vi "Write_raw_block_header.vi"(2 "Block Timings":T1, 3 "No of PWA samples":i32, 4 "Add to Block Header":string) -> (5 "Output string":string)   [LabVIEW 2020]
uses:
  Globals/Meas_global.vi
  Globals/Plug_in_data_global.vi
  Controls/Block_start_and_end.ctl
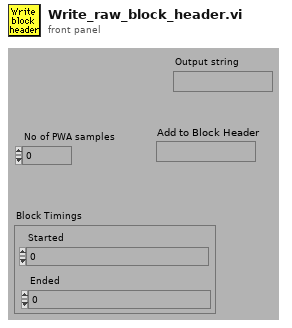
[diagram p1: front panel]
types:
  T1 = typedef "Block_start_and_end.ctl" = cluster{"Started":dbl, "Ended":dbl}
  T2 = typedef "Ch_description_ADAM.ctl" = cluster{"Ch Name":string, "Type":T3, "Function":T4, "Ch State":T5, "Calibration type":T6, "A":dbl, "B":dbl, "C":dbl, "D":dbl, "Comments":string, "Address":T7, "String":string, "Duty":u16}
  T3 = typedef "Module_type_ADAM.ctl" = string
  T4 = typedef "Function_ADAM.ctl" = enum16{"Analogue Input", "Digital Input", "Event counter", "Event rate", "Analogue Output", "Digital Output", "Relay Output"}
  T5 = typedef "Channel_State.ctl" = enum16{"On", "Off", "Always On", "Always Off"}
  T6 = typedef "Calib_type_ADAM.ctl" = string
  T7 = typedef "Address.ctl" = cluster{"Main":i32, "Ch.":i32, "Sub":i32, "Port Name":string}
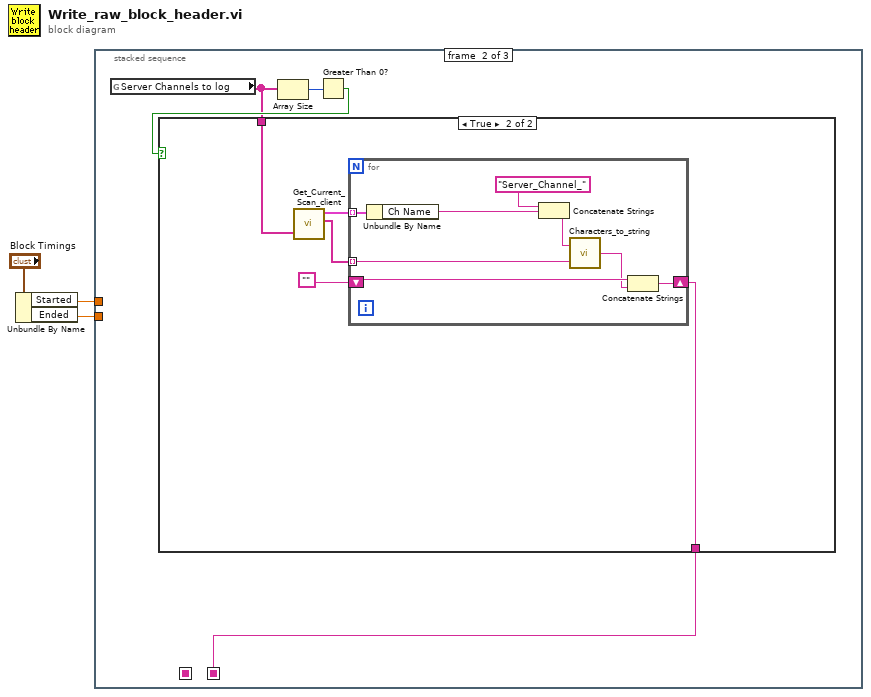
[diagram p0: block diagram]
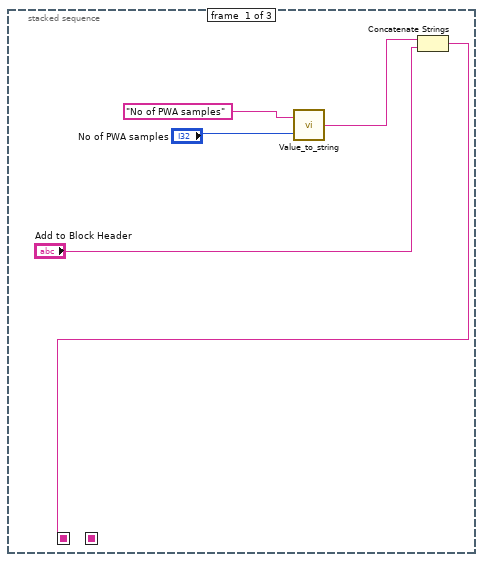
[diagram p2: hidden frame]
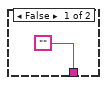
[diagram p3: hidden frame]
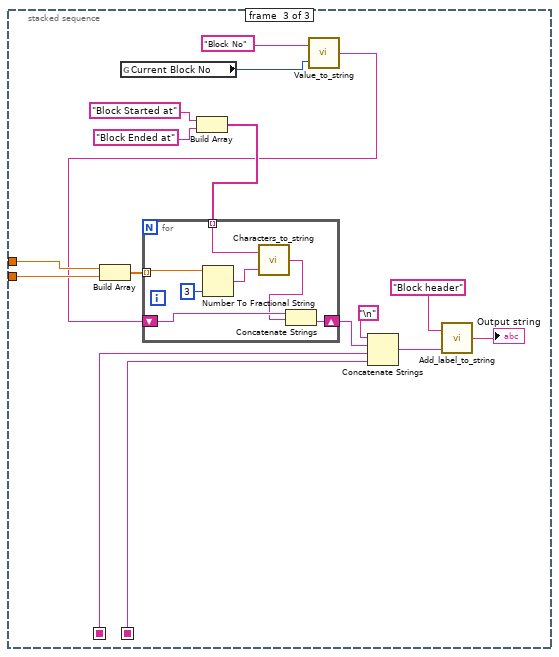
[diagram p4: hidden frame]
diagram:
  n1 = Unbundle By Name("Block Timings") -> ("Started"=w2:dbl, "Ended"=w1:dbl)
  n2 = stacked-sequence {
    seq-local: [w8 _ _] -> [_ _ w41]
    seq-local: [_ w9 _] -> [_ _ w28]
    tunnel: w2 -> [_ _ w34]
    tunnel: w1 -> [_ _ w33]
    frame #0 {
      n3 = call "Value_to_string.vi"("Value"="No of PWA samples", "Label for value"="No of PWA samples") -> ("Output string"=w5:string)  [unwired: 1 in]
      n4 = Concatenate Strings(w5, "Add to Block Header") -> (w8:string)
    }
    frame #1 {
      n5 = global read "Plug_in_data_global.vi" "Server Channels to log"() -> (w10:string[])
      n6 = Array Size(array=w10) -> (size(s)=w12:i32)
      n7 = Greater Than 0?(x=w12) -> (x > 0?=w11:bool)
      n8 = case shown="True" w11 {
        tunnel: w10 -> [_ w17]
        tunnel: ["" w14] -> w9
        frame False {
        }
        frame True {
          n9 = call "Get_Current_Scan_client.vi"("multipleChannels"=w17) -> ("Ch Description Array"=w16:T2[], "String values"=w15:string[])  [unwired: 2 in, 1 out]
          n10 = for {
            shift-right: [w25] -> w14
            shift-left: "" -> [w24]
            tunnel: w16 -> [w21] mode=indexing
            tunnel: w15 -> [w19] mode=indexing
            n11 = Unbundle By Name(w21) -> ("Ch Name"=w20:string)
            n12 = Concatenate Strings("Server_Channel_" ("string"), w20) -> (w22:string)
            n13 = call "Characters_to_string.vi"("Characters to write"=w19, "Label for characters"=w22) -> ("Output string"=w23:string)  [unwired: 1 in]
            n14 = Concatenate Strings(w24, w23) -> (w25:string)
          }
        }
      }
    }
    frame #2 {
      n15 = Build Array(w34, w33) -> (w35:dbl[])
      n16 = global read "Meas_global.vi" "Current Block No"() -> (w27:i32)
      n17 = Build Array("Block Started at", "Block Ended at") -> (w37:string[])
      n18 = call "Value_to_string.vi"("Value"=w27, "Label for value"="Block No") -> ("Output string"=w31:string)  [unwired: 1 in]
      n19 = for {
        tunnel: w37 -> [w49] mode=indexing
        shift-right: [w46] -> w39
        shift-left: w31 -> [w48]
        tunnel: w35 -> [w44] mode=indexing
        n20 = Number To Fractional String(number=w44, precision (6)=i16 3) -> (F-format string=w43:string)  [unwired: 2 out]
        n21 = call "Characters_to_string.vi"("Characters to write"=w43, "Label for characters"=w49) -> ("Output string"=w47:string)  [unwired: 1 in]
        n22 = Concatenate Strings(w48, w47) -> (w46:string)
      }
      n23 = Concatenate Strings("\n", w39, w41, w28) -> (w40:string)
      n24 = call "Add_label_to_string.vi"("String to write"=w40, "File Label"="Block header") -> ("Output string"=→"Output string":string)
    }
  }
